vi "ScanDelayStatus.vi"(8 "error in":errorcluster, 11 "VISA APE resource":refnum<visa-resource-name>) -> (0 "error out":errorcluster, 1 "new data":bool, 2 "status register":bool[](array[boolean]), 3 "error register":bool[](array[boolean])=[FALSE, FALSE, FALSE, FALSE, TRUE, FALSE, FALSE, FALSE], 4 "External trigger frequency (Hz)":dbl format="%.3f", 6 "reserved":bool[](array[boolean]))   [LabVIEW 2018]
uses:
  <vilib>/Instr/_visa.llb/Select Event Type.ctl
panel:
  # "Power amp active"
  # "Data acquisition trigger"
  # "Data acquisition active"
  # "External trigger detected"
  # "RESERVED"
  # "RESERVED"
  # "RESERVED"
  # "RESERVED"
  # "Parser error"
  # "Parameter error"
  # "FRAM error"
  # "I2C1 error"
  # "I2C2 error"
  # "RESERVED"
  # "RESERVED"
  # "RESERVED"
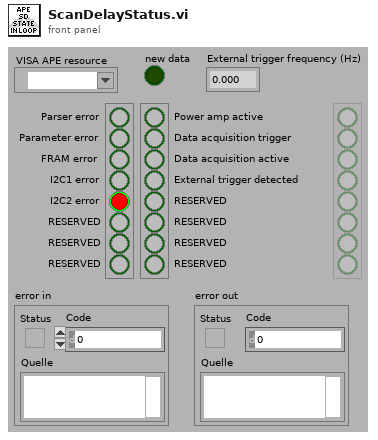
[diagram p1: front panel]
types:
  T1 = typedef "Select Event Type.ctl" = u32
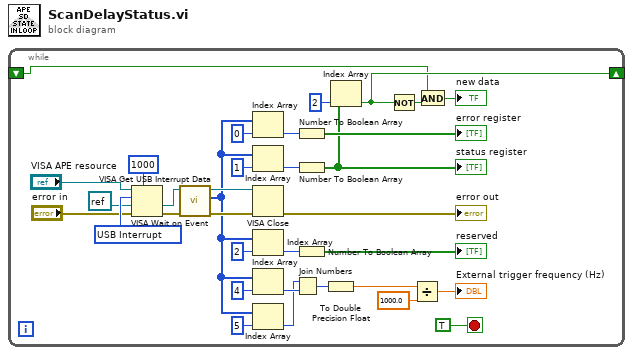
[diagram p0: block diagram]
diagram:
  n1 = while {
    shift-right: [w4] -> _
    shift-left: _ -> [w3]
    stop <- TRUE stop-if-true
    w17 = T1 1073684535 items=["Service Request"=1073684491, "Trigger"=3221168138, "Löschen"=1073684493, "VXI Signal"=1073684512, "VXI/VME Interrupt"=3221168161, "VXI/VME Sysfail"=1073684509, "VXI/VME Sysreset"=1073684510, "GPIB CIC"=1073684498, "GPIB Talk"=1073684499, "GPIB Listen"=1073684500, "PXI Interrupt"=1073684514, "Serial Break"=1073684515, "Serial TermChar"=1073684516, "Serial CTS"=1073684521, "Serial DSR"=1073684522, "Serial DCD"=1073684524, "Serial RI"=1073684526, "Serial Character"=1073684533, "USB Interrupt"=1073684535, "All Enabled"=1073709055] ("Event Type")
    n2 = VISA Wait on Event(7:u32 1000 ("timeout (0)"), 8:"error in", 9:refnum<visa-resource-name> refnum ("event class (Generic Event)"), 10:w17, 11:"VISA APE resource") -> (0:w13:errorcluster, 1:w12:refnum<visa-resource-name>)  [unwired: 2 out]
    n3 = call <vilib>:"VISA Get USB Interrupt Data.vi"("error in (no error)"=w13, "VISA USB Intr Event"=w12) -> ("error out"=w9:errorcluster, "data buffer"=w1:u8[], "VISA USB Intr Event out"=w10:refnum<visa-resource-name>)  [unwired: 7 out]
    n4 = Index Array(array=w1, index=0) -> (element=w20:u8)
    n5 = Index Array(array=w1, index=1) -> (element=w22:u8)
    n6 = VISA Close(VISA resource name=w10, error in (no error)=w9) -> (error out=→"error out":errorcluster)
    n7 = Index Array(array=w1, index=2) -> (element=w26:u8)
    n8 = Index Array(array=w1, index=4) -> (element=w30:u8)
    n9 = Index Array(array=w1, index=5) -> (element=w29:u8)
    n10 = Join Numbers(hi=w29, lo=w30) -> ((hi.lo)=w31:u16)
    n11 = Number To Boolean Array(number=w20) -> (Boolean array=→"error register":bool[])
    n12 = Number To Boolean Array(number=w22) -> (Boolean array=w6:bool[])
    "status register" <- w6
    n13 = Number To Boolean Array(number=w26) -> (Boolean array=→"reserved":bool[])
    n14 = To Double Precision Float(number=w31) -> (double precision float=w34:dbl)
    n15 = Index Array(array=w6, index=2) -> (element=w4:bool)
    n16 = Not(x=w4) -> (.not. x?=w5:bool)
    n17 = Divide(x=w34, y=1000.0) -> (x/y=→"External trigger frequency (Hz)":dbl)
    n18 = And(x=w3, y=w5) -> (x .and. y?=→"new data":bool)
  }
